vi "S-Curve - Tangent Semicircles.vi"() -> ()   [LabVIEW 2020]
panel:
  in  "End Amplitude":dbl
  in  "Number of Samples":i32 min=0
  out "Charge (mC)":dbl
  out "Waveform Graph":waveform(dbl)(graph)
  in  "Total Time (s)":dbl
  in  "Post-ramp\nRadius (s)":dbl
  in  "Pre-ramp\nRadius (s)":dbl
  in  "Start Amplitude":dbl
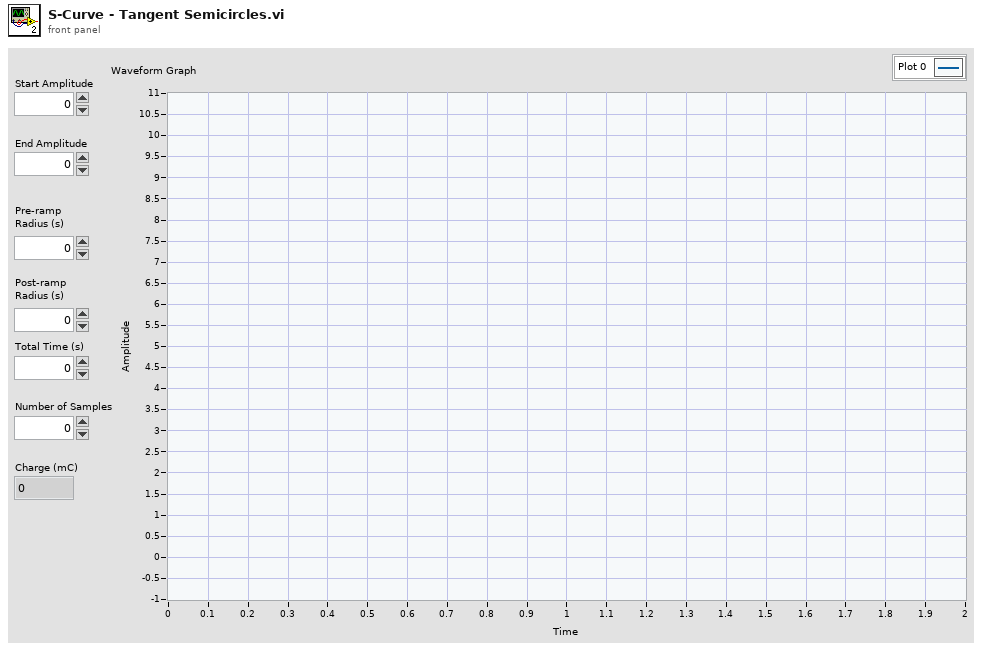
[diagram p1: front panel]
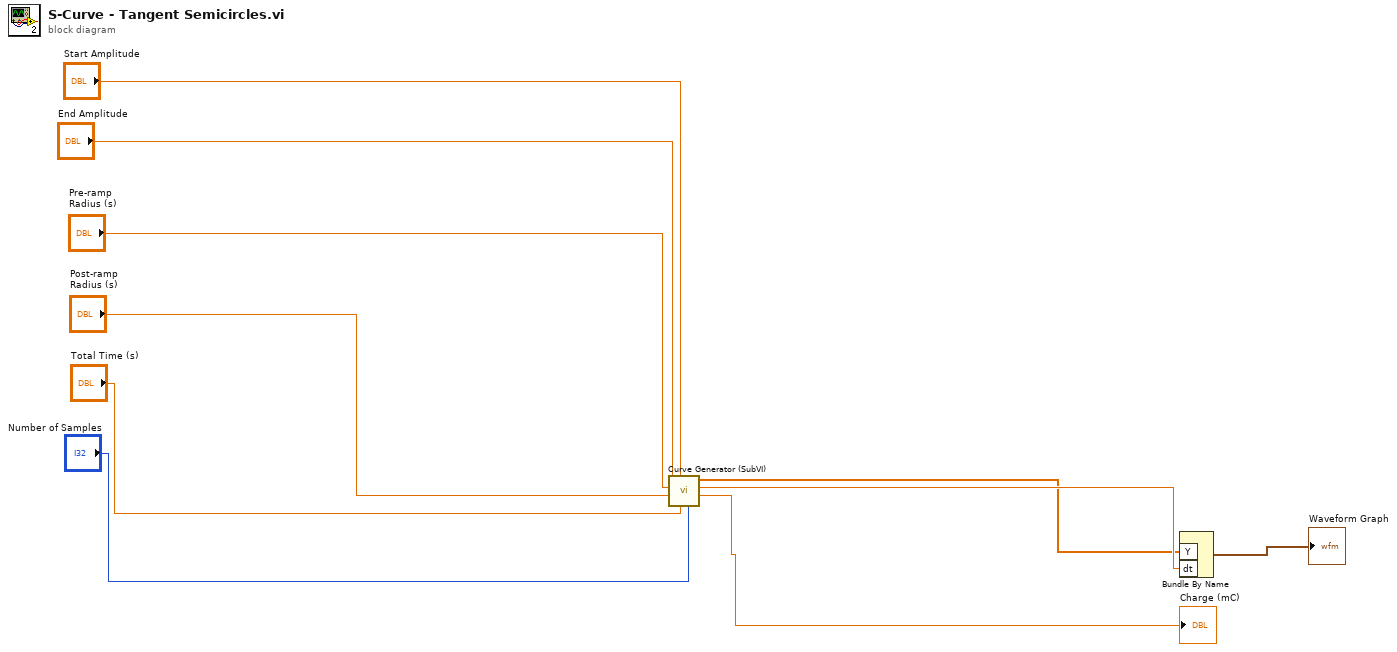
[diagram p0: block diagram]
diagram:
  n1 = call "Curve Generator (SubVI).vi"("Number of Samples"="Number of Samples", "Total Length (ms)"="Total Time (s)", "Start Amplitude (mA)"="Start Amplitude", "Post-ramp\nRadius (ms)"="Post-ramp\nRadius (s)", "Pre-ramp\nRadius (ms)"="Pre-ramp\nRadius (s)", "End Amplitude (mA)"="End Amplitude") -> ("Charge (mC)"=→"Charge (mC)":dbl, "dt"=w5:dbl, "S-Curve"=w3:dbl[])  [unwired: 3 in]
  n2 = Bundle By Name("Y"=w3, "dt"=w5) -> (→"Waveform Graph":waveform(dbl))  [unwired: 1 in]
